vi "create_data_header.vi"() -> (11 "String":string)   [LabVIEW 2016]
uses:
  Instrument_Setup.vi
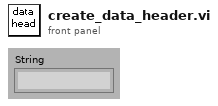
[diagram p1: front panel]
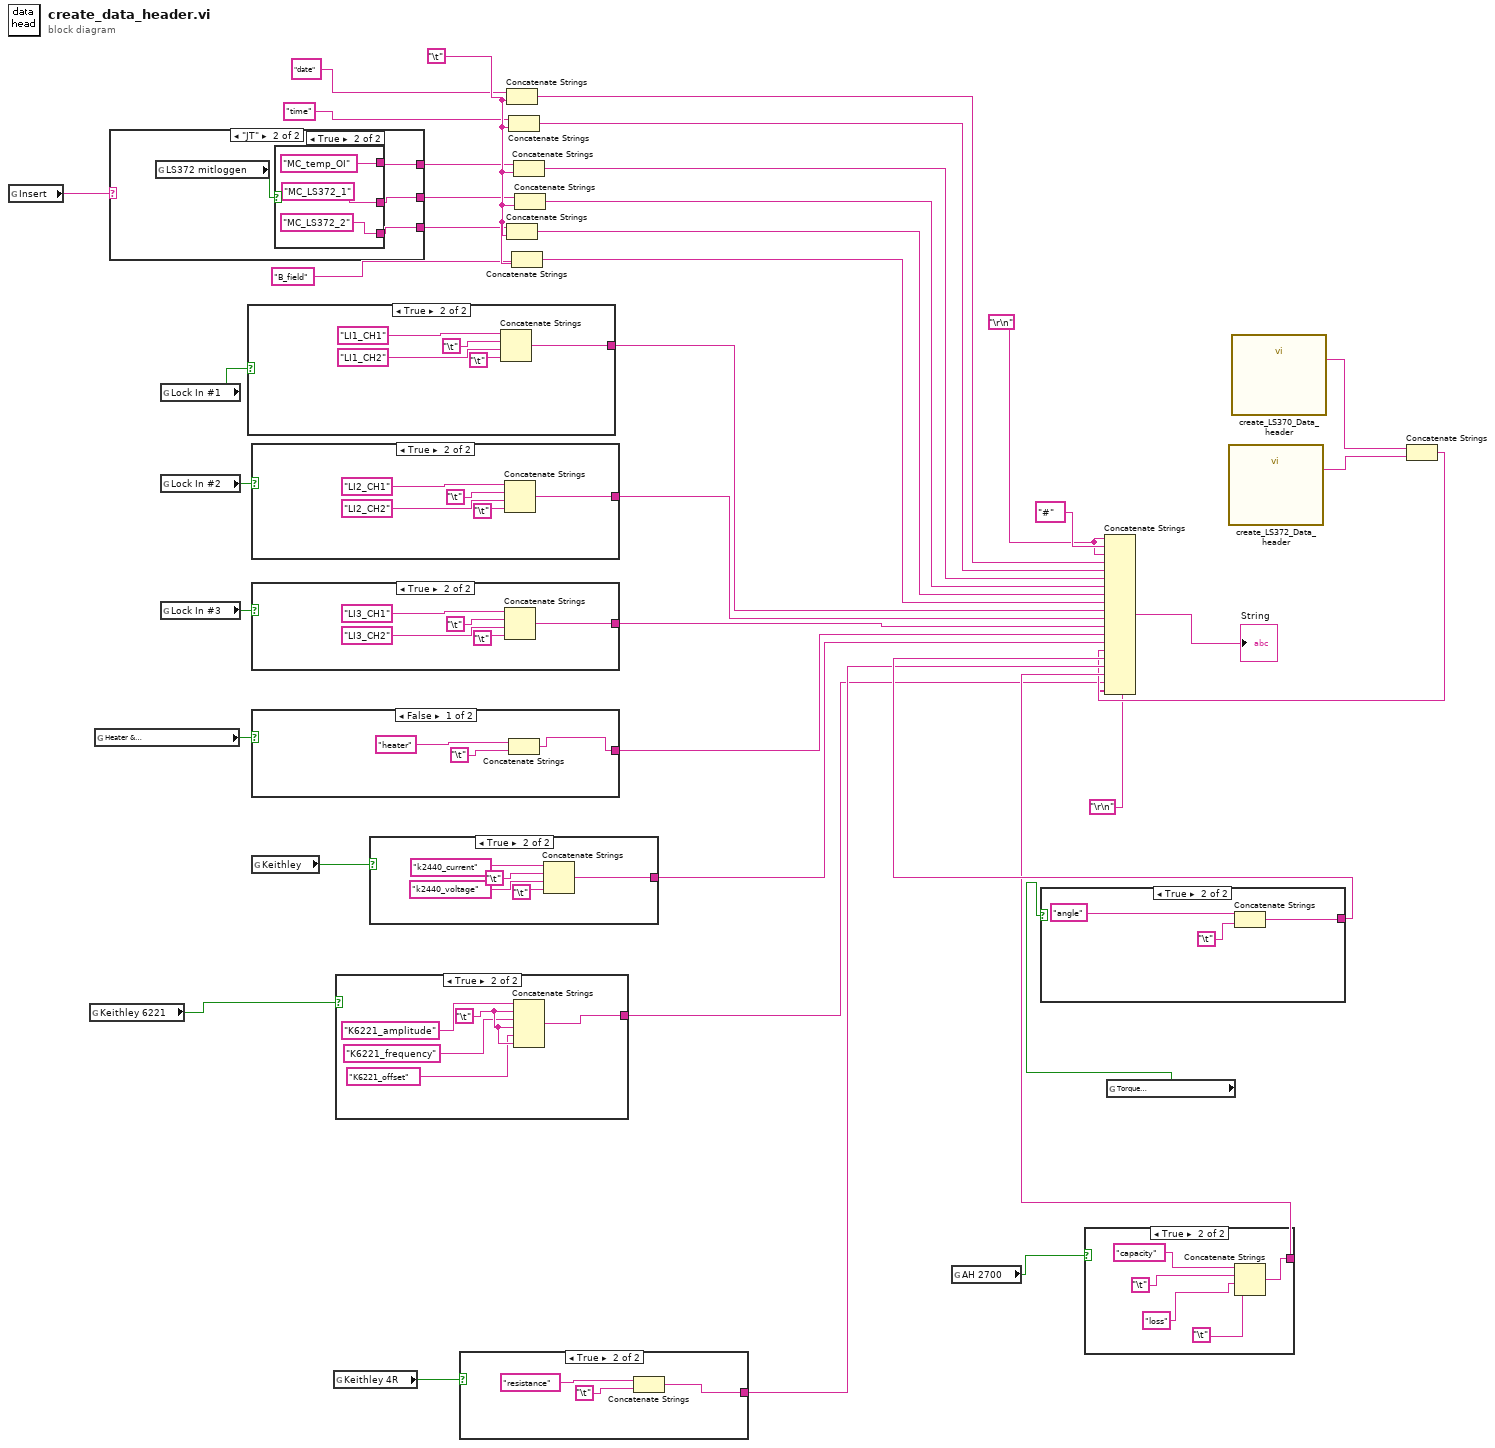
[diagram p0: block diagram]
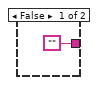
[diagram p2: hidden frame]
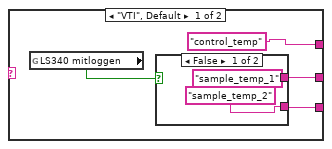
[diagram p3: hidden frame]
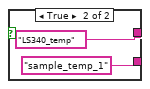
[diagram p4: hidden frame]
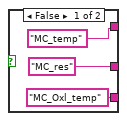
[diagram p5: hidden frame]
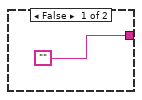
[diagram p6: hidden frame]
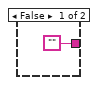
[diagram p7: hidden frame]
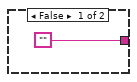
[diagram p8: hidden frame]
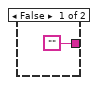
[diagram p9: hidden frame]
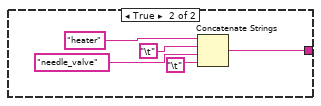
[diagram p10: hidden frame]
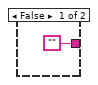
[diagram p11: hidden frame]
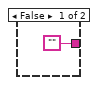
[diagram p12: hidden frame]
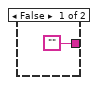
[diagram p13: hidden frame]
diagram:
  w27 = "\t"
  w10 = "\r\n"
  n1 = global read "Instrument_Setup.vi" "Insert"() -> (w13:string)
  n2 = global read "Instrument_Setup.vi" "Keithley 6221"() -> (w2:bool)
  n3 = global read "Instrument_Setup.vi" "Heater &\nNeedle Valve"() -> (w36:bool)
  n4 = case shown="\"JT\"" w13 {
    tunnel: ["control_temp" w51] -> w24
    tunnel: [w42 w50] -> w23
    tunnel: [w41 w49] -> w22
    frame "VTI", Default {
      n5 = global read "Instrument_Setup.vi" "LS340 mitloggen"() -> (w40:bool)
      n6 = case shown="False" w40 {
        tunnel: ["sample_temp_1" "LS340_temp"] -> w42
        tunnel: ["sample_temp_2" "sample_temp_1"] -> w41
        frame False {
        }
        frame True {
        }
      }
    }
    frame "JT" {
      n7 = global read "Instrument_Setup.vi" "LS372 mitloggen"() -> (w48:bool)
      n8 = case shown="True" w48 {
        tunnel: ["MC_temp" "MC_temp_OI"] -> w51
        tunnel: ["MC_res" "MC_LS372_1"] -> w50
        tunnel: ["MC_Oxl_temp" "MC_LS372_2"] -> w49
        frame False {
        }
        frame True {
        }
      }
    }
  }
  n9 = global read "Instrument_Setup.vi" "Lock In #1"() -> (w39:bool)
  n10 = global read "Instrument_Setup.vi" "Lock In #2"() -> (w38:bool)
  n11 = global read "Instrument_Setup.vi" "Lock In #3"() -> (w37:bool)
  n12 = case shown="True" w39 {
    tunnel: ["" w63] -> w34
    frame False {
    }
    frame True {
      n13 = Concatenate Strings("LI1_CH1", "\t", "LI1_CH2", "\t") -> (w63:string)
    }
  }
  n14 = case shown="True" w38 {
    tunnel: ["" w65] -> w33
    frame False {
    }
    frame True {
      n15 = Concatenate Strings("LI2_CH1", "\t", "LI2_CH2", "\t") -> (w65:string)
    }
  }
  n16 = case shown="True" w37 {
    tunnel: ["" w71] -> w32
    frame False {
    }
    frame True {
      n17 = Concatenate Strings("LI3_CH1", "\t", "LI3_CH2", "\t") -> (w71:string)
    }
  }
  n18 = case shown="False" w36 {
    tunnel: [w76 w83] -> w31
    frame False {
      n19 = Concatenate Strings("heater", "\t") -> (w76:string)
    }
    frame True {
      n20 = Concatenate Strings("heater", "\t", "needle_valve", "\t") -> (w83:string)
    }
  }
  n21 = global read "Instrument_Setup.vi" "Keithley"() -> (w35:bool)
  n22 = global read "Instrument_Setup.vi" "Keithley 4R"() -> (w28:bool)
  n23 = case shown="True" w2 {
    tunnel: ["" w89] -> w1
    frame False {
    }
    frame True {
      w87 = "\t"
      n24 = Concatenate Strings("K6221_amplitude", w87, "K6221_frequency", w87, "K6221_offset", w87) -> (w89:string)
    }
  }
  n25 = case shown="True" w35 {
    tunnel: ["" w95] -> w30
    frame False {
    }
    frame True {
      n26 = Concatenate Strings("k2440_current", "\t", "k2440_voltage", "\t") -> (w95:string)
    }
  }
  n27 = case shown="True" w28 {
    tunnel: ["" w99] -> w8
    frame False {
    }
    frame True {
      n28 = Concatenate Strings("resistance", "\t") -> (w99:string)
    }
  }
  n29 = Concatenate Strings("date", w27) -> (w15:string)
  n30 = Concatenate Strings(w22, w27) -> (w19:string)
  n31 = Concatenate Strings("time", w27) -> (w16:string)
  n32 = Concatenate Strings("B_field", w27) -> (w20:string)
  n33 = Concatenate Strings(w24, w27) -> (w17:string)
  n34 = Concatenate Strings(w23, w27) -> (w18:string)
  n35 = global read "Instrument_Setup.vi" "AH 2700"() -> (w12:bool)
  n36 = case shown="True" w12 {
    tunnel: ["" w102] -> w7
    frame False {
    }
    frame True {
      n37 = Concatenate Strings("capacity", "\t", "loss", "\t") -> (w102:string)
    }
  }
  n38 = global read "Instrument_Setup.vi" "Torque \nMeasurem."() -> (w29:bool)
  n39 = case shown="True" w29 {
    tunnel: ["" w109] -> w9
    frame False {
    }
    frame True {
      n40 = Concatenate Strings("angle", "\t") -> (w109:string)
    }
  }
  n41 = call "create_LS372_Data_header.vi"() -> ("String"=w5:string)  [unwired: 11 in]
  n42 = call "create_LS370_Data_header.vi"() -> ("String"=w6:string)  [unwired: 11 in]
  n43 = Concatenate Strings(w6, w5) -> (w4:string)
  n44 = Concatenate Strings(w10, "#", w10, w15, w16, w17, w18, w19, w20, w34, w33, w32, w31, w30, w4, w9, w8, w7, w1, "\r\n") -> (→"String":string)
